vi "CSP_updatePCA_Parameters.vi"(8 "error in (no error)":errorcluster, 10 "Indicators Ref":T1, 11 "CSP.lvclass in":refnum<class "CSP.lvclass">) -> (0 "error out":errorcluster, 3 "CSP.lvclass out":refnum<class "CSP.lvclass">)   [LabVIEW 2016, in "Spatial Pattern Filter.lvlib" / "CSP.lvclass"]
uses:
  CSP.lvclass
  CSP.lvclass/CSP.ctl
  Spatial Pattern Filter.lvlib
panel:
  # "This VI is a part of BCI Design library, http://www.ru-bci.org \nCopyright © 2020, Sotnikov Peter, All rights reserved. License: CC BY-NC 4.0"
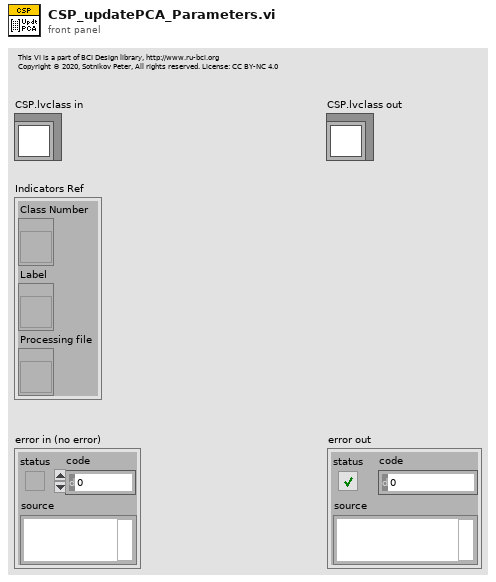
[diagram p1: front panel]
types:
  T1 = cluster{"Class Number":refnum<vi>, "Label":refnum<vi>, "Processing file":refnum<vi>}
  T2 = typedef "NI_Matrix.lvlib/RealMatrix.ctl" = dbl[][]
  T3 = cluster{"PCAMatrix":T2, "CovarianceMatrix":T2, "MeanValue":dbl[][]}[]
  T4 = cluster{"PCAMatrix":T2, "CovarianceMatrix":T2, "MeanValue":dbl[][]}
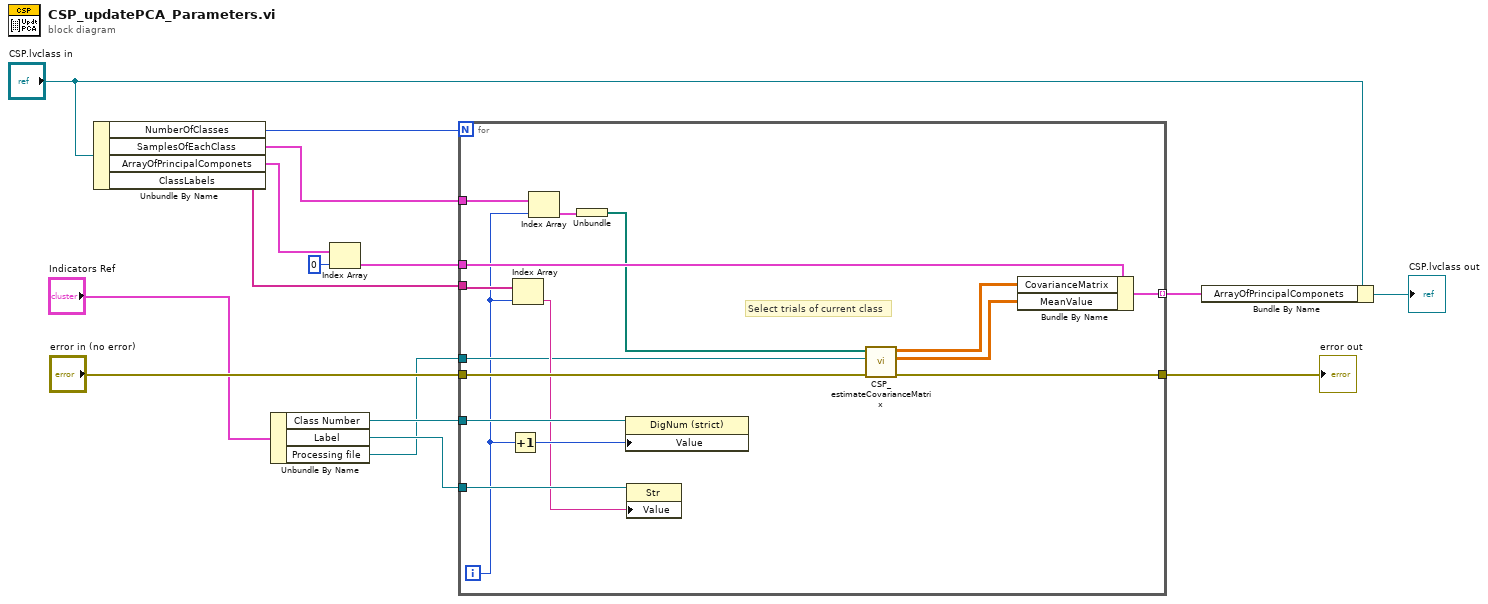
[diagram p0: block diagram]
diagram:
  n1 = Unbundle By Name("CSP.lvclass in") -> ("NumberOfClasses"=w14:i32, "SamplesOfEachClass"=w15:cluster{"ArrayOfFiles":path[]}[], "ArrayOfPrincipalComponets"=w10:T3, "ClassLabels"=w4:string[])
  n2 = Unbundle By Name("Indicators Ref") -> ("Class Number"=w5:refnum<vi>, "Label"=w3:refnum<vi>, "Processing file"=w2:refnum<vi>)
  n3 = Index Array(array=w10, index=0) -> (element=w8:T4)
  n4 = for {
    N: w14 -> [_]
    tunnel: w15 -> [w30]
    tunnel: [w31] -> w7 mode=indexing
    tunnel: "error in (no error)" -> [w29]
    tunnel: w8 -> [w28]
    tunnel: w5 -> [w27]
    tunnel: w4 -> [w25]
    tunnel: w3 -> [w24]
    tunnel: w2 -> [w22]
    tunnel: [w18] -> w1
    i -> [w21]
    # "Select trials of current class"
    n5 = Increment(x=w21) -> (x+1=w26:i32)
    n6 = Index Array(array=w25, index=w21) -> (element=w23:string)
    n7 = Index Array(array=w30, index=w21) -> (element=w17:cluster{"ArrayOfFiles":path[]})
    n8 = Unbundle(w17) -> ("ArrayOfFiles"=w16:path[])
    n9 = property class="DigNum (strict)"(reference=w27, "Value"=w26) -> ()  [unwired: 1 in, 2 out]
    n10 = property class="Str"(reference=w24, "Value"=w23) -> ()  [unwired: 1 in, 2 out]
    n11 = call "CSP_estimateCovarianceMatrix.vi"("error in (no error)"=w29, "Processing file"=w22, "FilePaths"=w16) -> ("error out"=w18:errorcluster, "Mean Trial"=w19:dbl[][], "Covariance Matrix"=w20:T2)  [unwired: 6 in]
    n12 = Bundle By Name(cluster=w28, "CovarianceMatrix"=w20, "MeanValue"=w19) -> (w31:T4)
  }
  "error out" <- w1
  n13 = Bundle By Name(cluster="CSP.lvclass in", "ArrayOfPrincipalComponets"=w7) -> (→"CSP.lvclass out":refnum<class "CSP.lvclass">)
